vi "Extract Received Data Set.vi"(8 "Error In":errorcluster, 11 "Received Array In":u8[](array[numeric]) format="%02x") -> (0 "Error Out":errorcluster, 1 "New Data Set Received":bool, 2 "Extracted Data Set":u8[](array[numeric]), 3 "Received Array Out":u8[](array[numeric]))   [LabVIEW 2012]
doc: "This VI extracts a single data set from a received data stream.\n\nThe extracted command is removed from the data stream.\n\nTBD. Use the checksum to validate that the whole packet has been read."
panel:
  out "Payload Length":u8 format="%02x"
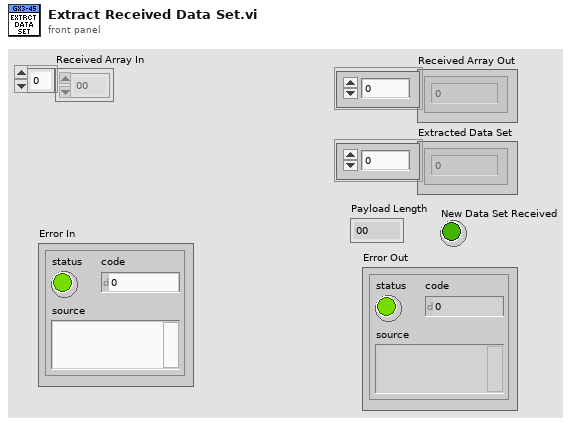
[diagram p1: front panel]
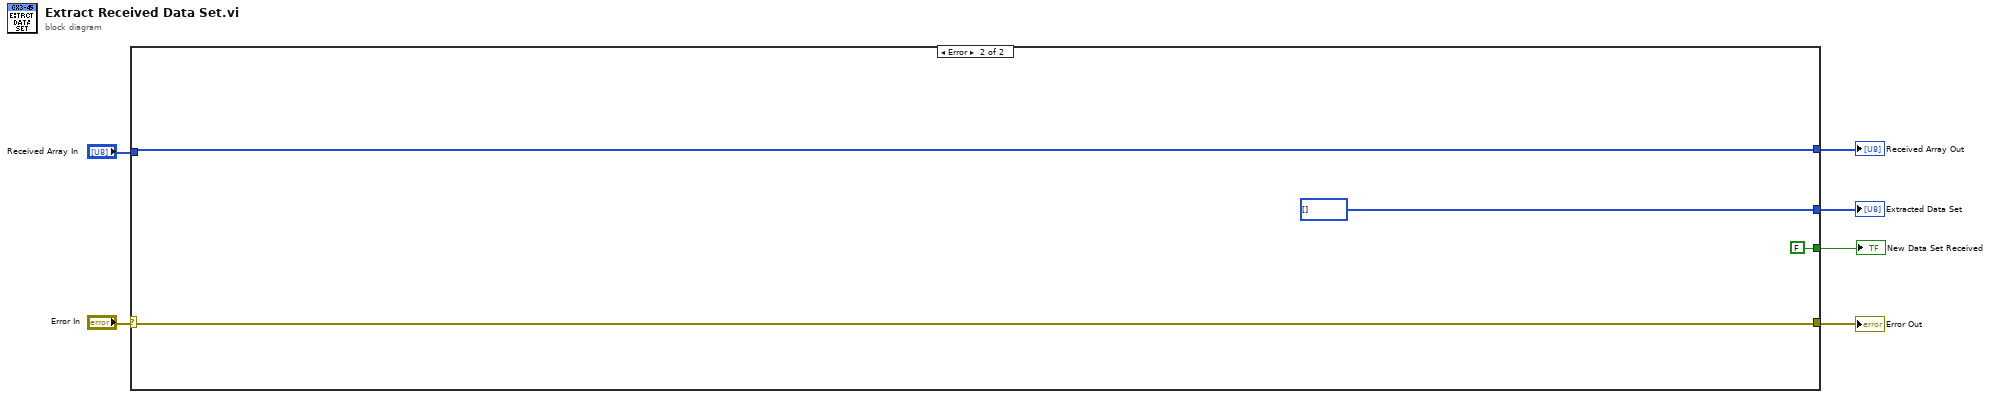
[diagram p0: block diagram]
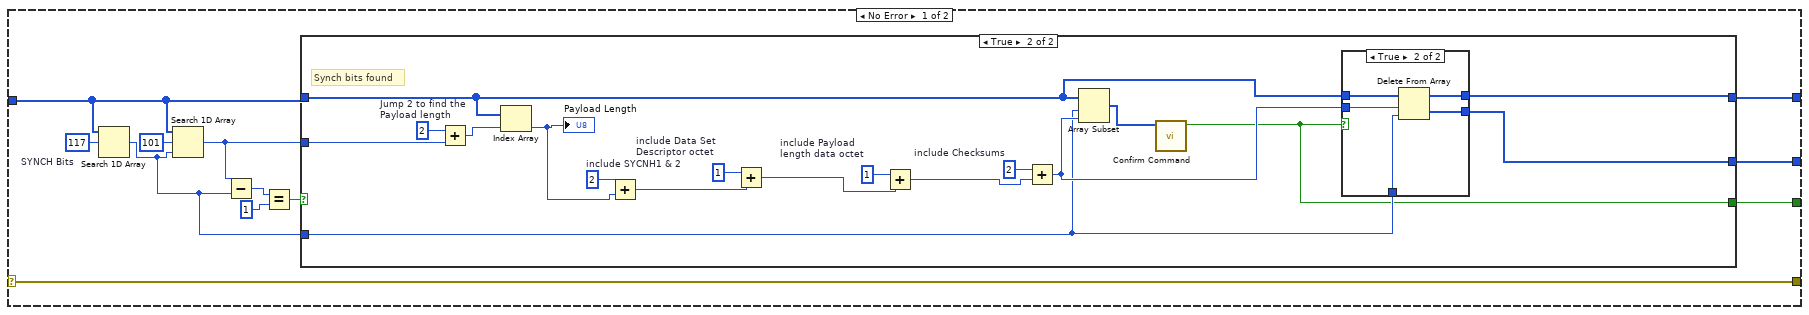
[diagram p2: hidden frame]
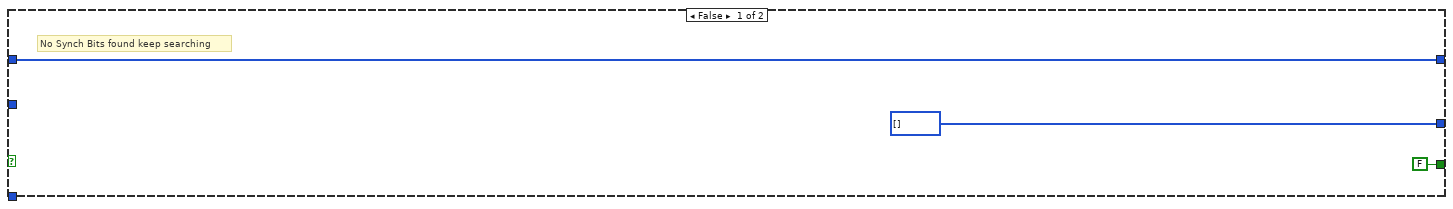
[diagram p3: hidden frame]
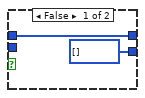
[diagram p4: hidden frame]
diagram:
  n1 = case shown="Error" "Error In" {
    selector: "Error In" -> [w8 w50]
    tunnel: "Received Array In" -> [w11 w49]
    tunnel: [w10 w49] -> w5
    tunnel: [w9 u8[] [] ("Received Array In")] -> w4
    tunnel: [w8 w50] -> w2
    tunnel: [w7 FALSE ("Full command received")] -> w1
    frame No Error {
      w18 = u8 117  # SYNCH Bits
      n2 = Search 1D Array(1D array=w11, element=w18) -> (index of element=w12:i32)  [unwired: 1 in]
      n3 = Search 1D Array(1D array=w11, element=u8 101, start index (0)=w12) -> (index of element=w13:i32)
      n4 = Subtract(x=w13, y=w12) -> (x-y=w16:i32)
      n5 = Equal?(x=w16, y=1) -> (x = y?=w14:bool)
      n6 = case shown="True" w14 {
        tunnel: w13 -> [_ w38]
        tunnel: w11 -> [w21 w26]
        tunnel: w12 -> [_ w23]
        tunnel: [w21 w25] -> w10
        tunnel: [u8[] [] ("Received Array In") w27] -> w9
        tunnel: [FALSE ("Full command received") w22] -> w7
        frame False {
          # "No Synch Bits found keep searching"
        }
        frame True {
          w31 = 1  # include Payload  length data octet
          w34 = 1  # include Data Set  Descriptor octet
          w35 = 2  # include SYCNH1 & 2
          w36 = 2  # include Checksums
          w39 = 2  # Jump 2 to find the  Payload length
          # "Synch bits found"
          n7 = Add(x=w39, y=w38) -> (x+y=w37:i32)
          n8 = Index Array(array=w26, index=w37) -> (element=w33:u8)
          "Payload Length" <- w33
          n9 = Add(x=w35, y=w33) -> (x+y=w32:i32)
          n10 = Add(x=w34, y=w32) -> (x+y=w30:i32)
          n11 = Add(x=w31, y=w30) -> (x+y=w29:i32)
          n12 = Add(x=w36, y=w29) -> (x+y=w24:i32)
          n13 = Array Subset(array=w26, index=w23, length=w24) -> (w28:u8[])
          n14 = call "Confirm Command.vi"("Extracted Data Set"=w28) -> ("Full command received"=w22:bool)  [unwired: 10 in]
          n15 = case shown="True" w22 {
            tunnel: [u8[] [] ("Received Array In") w46] -> w27
            tunnel: w26 -> [w41 w45]
            tunnel: [w41 w44] -> w25
            tunnel: w24 -> [_ w43]
            tunnel: w23 -> [_ w42]
            frame False {
            }
            frame True {
              n16 = Delete From Array(array=w45, length=w43, index=w42) -> (deleted portion=w46:u8[], array with subset deleted=w44:u8[])
            }
          }
        }
      }
    }
    frame Error {
    }
  }
  "Received Array Out" <- w5
  "Extracted Data Set" <- w4
  "Error Out" <- w2
  "New Data Set Received" <- w1
